vi "Calc Max Width And Height.vi"(9 "Point 3":T1, 10 "Point 2":T1, 11 "Point 1":T1) -> (2 "Max Width":i32, 3 "Max Height":i32)   [LabVIEW 2022 SP3, in "Raster.lvlib"]
uses:
  Raster.lvlib
  Point 2D.ctl
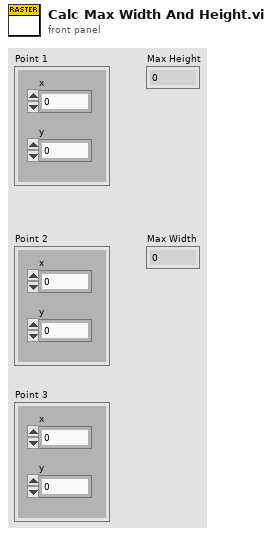
[diagram p1: front panel]
types:
  T1 = typedef "Raster.lvlib/Point 2D.ctl" = cluster{"x":i32, "y":i32}
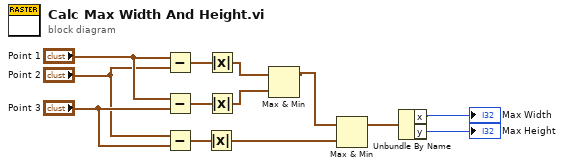
[diagram p0: block diagram]
diagram:
  n1 = Subtract(x="Point 1", y="Point 2") -> (x-y=w10:T1)
  n2 = Subtract(x="Point 1", y="Point 3") -> (x-y=w9:T1)
  n3 = Subtract(x="Point 2", y="Point 3") -> (x-y=w8:T1)
  n4 = Absolute Value(x=w8) -> (abs(x)=w4:T1)
  n5 = Absolute Value(x=w10) -> (abs(x)=w7:T1)
  n6 = Absolute Value(x=w9) -> (abs(x)=w6:T1)
  n7 = Max & Min(x=w7, y=w6) -> (max(x,y)=w5:T1)  [unwired: 1 out]
  n8 = Max & Min(x=w5, y=w4) -> (max(x,y)=w3:T1)  [unwired: 1 out]
  n9 = Unbundle By Name(w3) -> ("x"=→"Max Width":i32, "y"=→"Max Height":i32)
